vi "SVL Limit Testing (waveform).vi"(8 "error in (no error)":errorcluster, 9 "lower limit":cluster{"x0":dbl, "dx":dbl, "Y":dbl[]}={"x0"=0.0, "dx"=1.0, "Y"=[]} {"Y" format="%.2f"; "dx" format="%.2f"; "x0" format="%.2f"}, 10 "upper limit":cluster{"x0":dbl, "dx":dbl, "Y":dbl[]}={"x0"=0.0, "dx"=1.0, "Y"=[]} {"Y" format="%.2f"; "dx" format="%.2f"; "x0" format="%.2f"}, 11 "signal in":waveform(dbl)) -> (0 "error out":errorcluster, 1 "output values":waveform(dbl)[](graph), 2 "test results":bool[](array[boolean]), 3 "test passed?":bool)   [LabVIEW 2017, in "SoundVib_LimitTest.lvlib"]
doc: "Performs limit testing on waveforms, spectra, XY data, identified peaks, or scalar measurements. You can specify an upper and lower boundary of the envelope to define a pass range. This VI uses the defined pass range to test the input signal. VI outputs apply only to the current input signal. You can wire output values to a graph to view the limits, signal, and failures. Wire data to the<B> signal in</B> input to determine the polymorphic instance to use or manually select the instance."
uses:
  <vilib>/addons/Sound and Vibration/svt_Limit Test/SoundVib_LimitTest.lvlib
  <vilib>/measure/NI_MAPro.lvlib
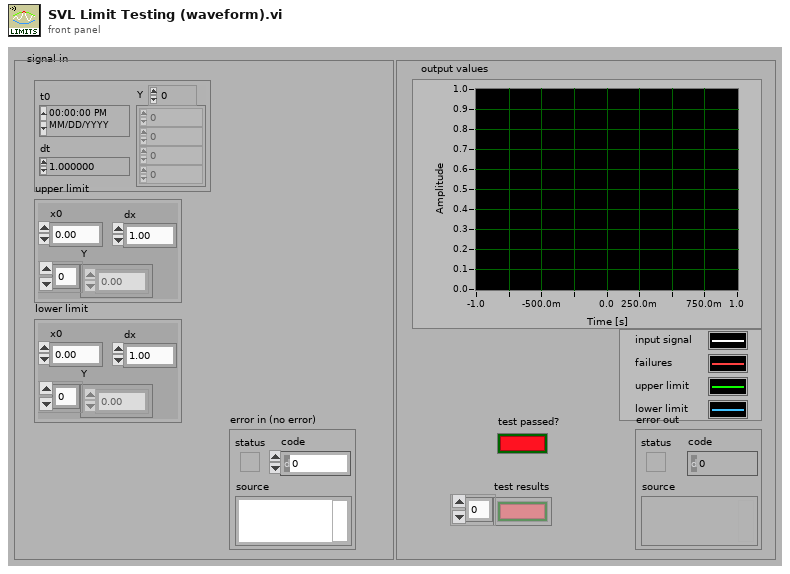
[diagram p1: front panel]
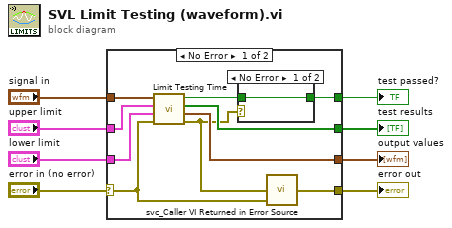
[diagram p0: block diagram]
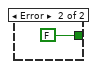
[diagram p2: hidden frame]
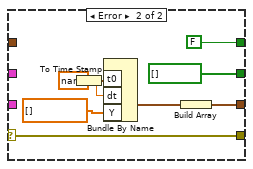
[diagram p3: hidden frame]
diagram:
  n1 = case shown="No Error" "error in (no error)" {
    selector: "error in (no error)" -> [w9 w28]
    tunnel: "signal in" -> [w18 _]
    tunnel: "upper limit" -> [w17 _]
    tunnel: "lower limit" -> [w16 _]
    tunnel: [w11 FALSE ("test passed?")] -> w5
    tunnel: [w15 bool[] [] ("test results")] -> w4
    tunnel: [w14 w22] -> w3
    tunnel: [w13 w28] -> w2
    frame No Error {
      n2 = call <vilib>:"Limit Testing Time.vi"("error in (no error)"=w9, "lower limit"=w16, "upper limit"=w17, "signal in"=w18) -> ("error out"=w10:errorcluster, "output values"=w14:waveform(dbl)[], "test results"=w15:bool[], "test passed?"=w12:bool)  [unwired: 2 in, 2 out]
      n3 = case shown="No Error" w10 {
        tunnel: w12 -> [w19 _]
        tunnel: [w19 FALSE ("test passed?")] -> w11
        frame No Error {
        }
        frame Error {
        }
      }
      n4 = call <vilib>:"svc_Caller VI Returned in Error Source.vi"("warning input to caller"=w9, "error in (no error)"=w10) -> ("error out"=w13:errorcluster)  [unwired: 3 in]
    }
    frame Error {
      w25 = nan ("t0")
      n5 = To Time Stamp(1:w25) -> (0:w21:timestamp)
      n6 = Bundle By Name("t0"=w21, "dt"=w25, "Y"=dbl[] []) -> (w23:waveform(dbl))  [unwired: 1 in]
      n7 = Build Array(w23) -> (w22:waveform(dbl)[])
    }
  }
  "test passed?" <- w5
  "test results" <- w4
  "output values" <- w3
  "error out" <- w2
